vi "Untitled 1.vi"() -> ()   [LabVIEW 2020]
panel:
  out "output 1":dbl
  out "after substring":string
  out "match substring":string
  out "before substring":string
  out "offset past match":i32
  in  "input 2":dbl
  out "Longitud":i32
  in  "Unidades":string="Volts"
  in  "Encabezado":string="El valor de voltaje es: "
  out "concatenated string":string
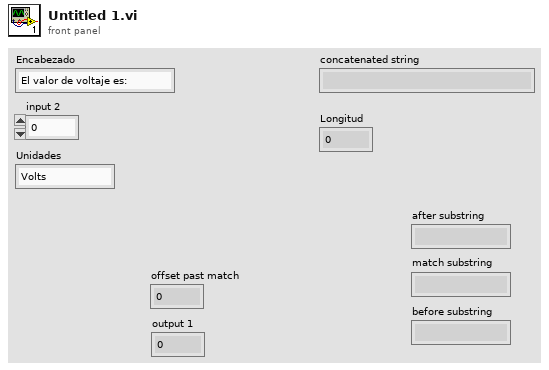
[diagram p1: front panel]
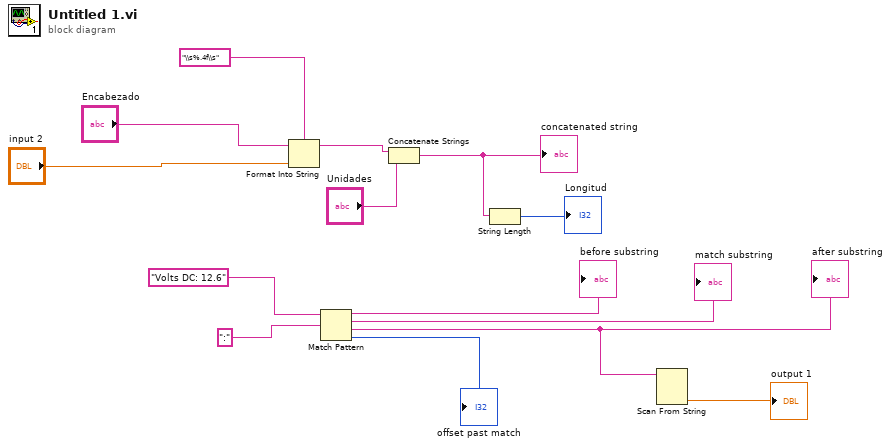
[diagram p0: block diagram]
diagram:
  n1 = Format Into String "Format Into String"(format string="\\s%.4f\\s", initial string="Encabezado", "input 2") -> (resulting string=w10:string)  [unwired: 1 in, 1 out]
  n2 = Match Pattern(string="Volts DC: 12.6", regular expression=":") -> (before substring=→"before substring":string, match substring=→"match substring":string, after substring=w1:string, offset past match=→"offset past match":i32)  [unwired: 1 in]
  "after substring" <- w1
  n3 = Concatenate Strings "Concatenate Strings"(w10, "Unidades") -> (w9:string)
  "concatenated string" <- w9
  n4 = String Length(string=w9) -> (length=→"Longitud":i32)
  n5 = Scan From String "Scan From String"(input string=w1) -> (output 1=→"output 1":dbl)  [unwired: 4 in, 3 out]
